vi "SetSmplDepth.vi"(8 "错误输入（无错误）":errorcluster, 10 "采样深度":u16) -> (0 "错误输出":errorcluster)   [LabVIEW 2018]
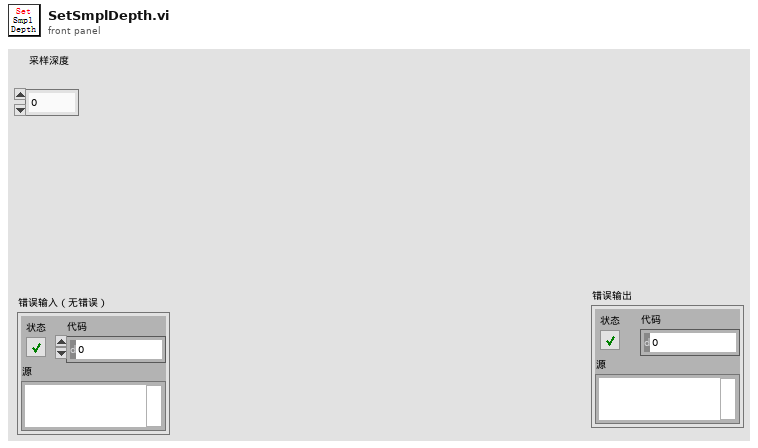
[diagram p1: front panel]
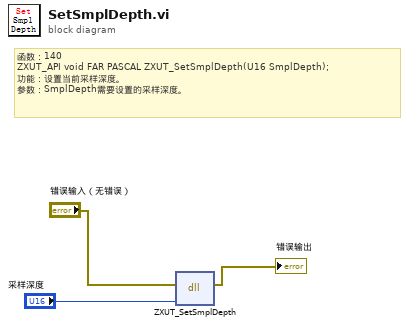
[diagram p0: block diagram]
diagram:
  # "函数：140\nZXUT_API void\tFAR PASCAL ZXUT_SetSmplDepth(U16 SmplDepth);\n功能：设置当前采样深度。\n参数：SmplDepth需要设置的采样深度。"
  n1 = dll-call lib="PTH2Rabs E软件项目超声超声子VI函数VI\tTCG处理ZXUTConfigMgr.dll" fn="ZXUT_SetSmplDepth"(error in="错误输入（无错误）", "SmplDepth"="采样深度") -> (error out=→"错误输出":errorcluster)  [unwired: 4 in, 1 out]
